vi "Expand Target Groups.vi"(6 "Cluster":refnum<class "Cluster Config.lvclass">, 7 "VolatusAPI":refnum<class "VolatusAPI.lvclass">, 8 "error in (no error)":errorcluster, 10 "Target Names":string[](array[string])) -> (0 "error out":errorcluster, 2 "Nodes":string[](array[string]))   [LabVIEW 2020, in "VolatusGUIElements.lvlib" / "LoggingControl.lvclass"]
uses:
  LoggingControl.lvclass
  LoggingControl.lvclass/LoggingControl.ctl
  Volatus/VolatusAPI/VolatusAPI.lvclass
  VolatusConfig/Cluster/Cluster Config.lvclass
  VolatusConfig/VolatusConfigElement/VolatusConfigElement.lvclass
  VolatusErrorUtilities/MultiErrors/MultiErrors.lvclass
  VolatusConfig/Node/Node Config.lvclass
  C:/dev/lv20CE/relink/lv-volatus/VolatusConfig/VolatusConfigElement/VolatusConfigElement.lvclass
  C:/dev/lv20CE/relink/lv-volatus/VolatusConfig/Node/Node Config.lvclass
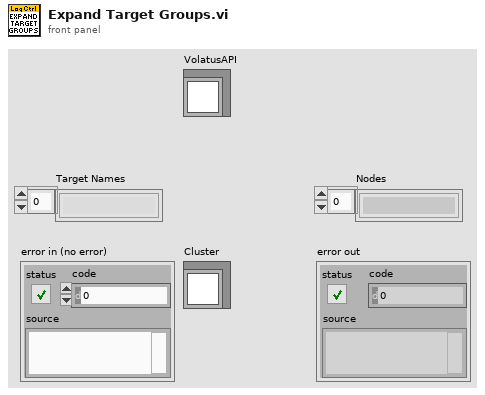
[diagram p1: front panel]
types:
  T1 = typedef "VolatusConfig.lvlib/Target Type.ctl" = enum16{"Unknown", "Node", "Group"}
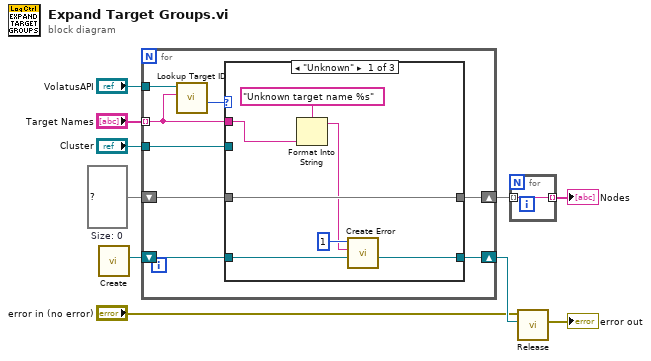
[diagram p0: block diagram]
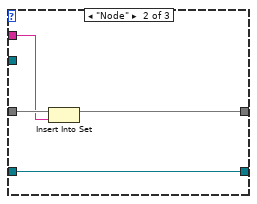
[diagram p2: hidden frame]
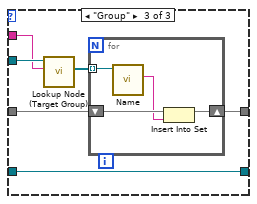
[diagram p3: hidden frame]
diagram:
  w8 = set{string} {}  # Size: 0
  n1 = call "Create.vi"() -> ("MultiErrors out"=w4:refnum<class "MultiErrors.lvclass">)  [unwired: 11 in]
  n2 = for {
    tunnel: "Target Names" -> [w16] mode=indexing
    tunnel: "VolatusAPI" -> [w18]
    shift-right: [w14] -> w6
    shift-left: w8 -> [w15]
    tunnel: "Cluster" -> [w13]
    shift-right: [w11] -> w3
    shift-left: w4 -> [w12]
    n3 = call "Lookup Target ID.vi"("Target Name"=w16, "VolatusAPI in"=w18) -> ("Type"=w17:T1)  [unwired: 6 in, 3 out]
    n4 = case shown="\"Unknown\"" w17 {
      tunnel: w16 -> [w20 w28 w34]
      tunnel: w15 -> [w25 w29 w32]
      tunnel: [w25 w27 w31] -> w14
      tunnel: w13 -> [_ _ w35]
      tunnel: w12 -> [w24 w26 w30]
      tunnel: [w23 w26 w30] -> w11
      frame "Unknown" {
        n5 = Format Into String(format string="Unknown target name %s", w20) -> (resulting string=w19:string)  [unwired: 2 in, 1 out]
        n6 = call "Create Error.vi"("MultiErrors in"=w24, "Message"=w19, "Code"=1) -> ("MultiErrors out"=w23:refnum<class "MultiErrors.lvclass">)  [unwired: 8 in]
      }
      frame "Node" {
        n7 = Insert Into Set(10:w28, 11:w29) -> (3:w27:set{string})  [unwired: 1 out]
      }
      frame "Group" {
        n8 = call "Lookup Node (Target Group).vi"("Target Name"=w34, "Cluster in"=w35) -> ("Nodes"=w33:refnum<class "Node Config.lvclass">[])  [unwired: 7 in, 2 out]
        n9 = for {
          tunnel: w33 -> [w39] mode=indexing
          shift-right: [w36] -> w31
          shift-left: w32 -> [w38]
          n10 = call "Name.vi"("VolatusConfigElement in"=w39) -> ("Name"=w37:string)  [unwired: 8 in, 2 out]
          n11 = Insert Into Set(10:w37, 11:w38) -> (3:w36:set{string})  [unwired: 1 out]
        }
      }
    }
  }
  n12 = for {
    tunnel: [w40] -> w7 mode=indexing
    tunnel: w6 -> [w40] mode=indexing
  }
  "Nodes" <- w7
  n13 = call "Release.vi"("MultiErrors in"=w3, "Upstream Error (None)"="error in (no error)") -> ("error out"=→"error out":errorcluster)  [unwired: 9 in]
